vi "GetSubVIReference.vi"(8 "error in":errorcluster, 11 "SubVI in":refnum<class "SubVI.lvclass">) -> (0 "error out":errorcluster, 1 "SubVI reference":refnum<vi>, 3 "SubVI out":refnum<class "SubVI.lvclass">)   [LabVIEW 2014, in "Raspberry Pi Compatible Compiler for LabVIEW.lvlib" / "SubVI.lvclass"]
uses:
  SubVI.lvclass
  Generic/Generic.lvclass
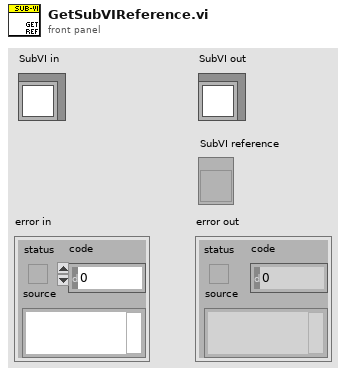
[diagram p1: front panel]
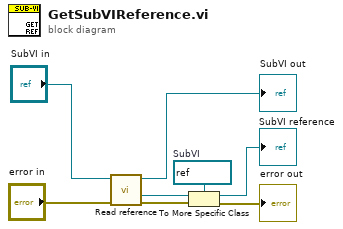
[diagram p0: block diagram]
diagram:
  w4 = refnum<vi> refnum  # SubVI
  n1 = call "Read reference.vi"("error in"="error in", "GObject in"="SubVI in") -> ("error out"=w6:errorcluster, "reference"=w2:refnum<vi>, "GObject out"=→"SubVI out":refnum<class "SubVI.lvclass">)  [unwired: 5 in]
  n2 = To More Specific Class(target class=w4, reference=w2, error in=w6) -> (specific class reference=→"SubVI reference":refnum<vi>, error out=→"error out":errorcluster)
